vi "Page_Info_Initialize.vi"(8 "error in (no error)":errorcluster, 9 "ctlReferences":T1, 11 "AB_SourceDistribution in":refnum<class "AB_SourceDistribution.lvclass">) -> (0 "error out":errorcluster, 3 "AB_SourceDistribution out":refnum<class "AB_SourceDistribution.lvclass">)   [LabVIEW 2020, in "AB_SourceDistribution.lvclass"]
uses:
  <vilib>/AppBuilder/AB_Classes/SourceDistribution/AB_SourceDistribution.lvclass
  <resource>/Framework/Providers/Builds/AppBuilder/AB_UI_Page_Info_References.ctl
  <resource>/Framework/Providers/Common/provcom_StringGlobals.vi
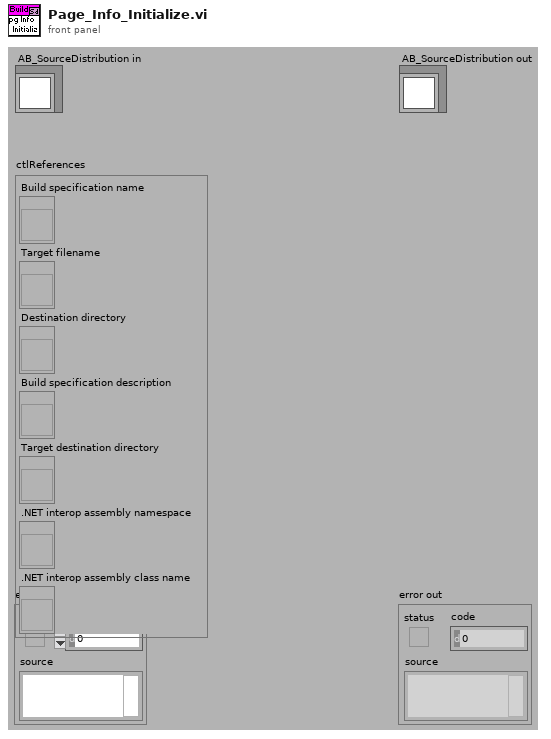
[diagram p1: front panel]
types:
  T1 = typedef "AB_UI_Page_Info_References.ctl" = cluster{"Build specification name":refnum<vi>, "Target filename":refnum<vi>, "Destination directory":refnum<vi>, "Build specification description":refnum<vi>, "Target destination directory":refnum<vi>, ".NET interop assembly namespace":refnum<vi>, ".NET interop assembly class name":refnum<vi>}
  T2 = typedef "LVRectTypeDef.ctl" = cluster{"Left":i16, "Top":i16, "Right":i16, "Bottom":i16}
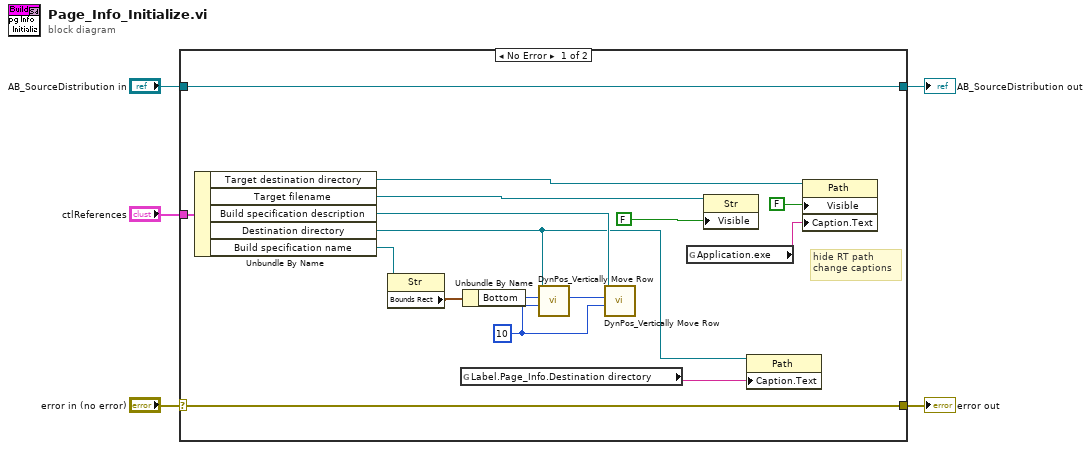
[diagram p0: block diagram]
diagram:
  n1 = case shown="No Error" "error in (no error)" {
    selector: "error in (no error)" -> [w19 w23]
    tunnel: [w19 w23] -> w4
    tunnel: [w20 w22] -> w2
    tunnel: "AB_SourceDistribution in" -> [w20 w22]
    tunnel: "ctlReferences" -> [w21 _]
    frame No Error {
      w14 = 10 ("Pixel separation (6)")
      # "hide RT path\nchange captions"
      n2 = Unbundle By Name(w21) -> ("Target destination directory"=w9:refnum<vi>, "Target filename"=w12:refnum<vi>, "Build specification description"=w13:refnum<vi>, "Destination directory"=w6:refnum<vi>, "Build specification name"=w17:refnum<vi>)
      n3 = property class="Str"(reference=w17) -> ("Bounds Rect"=w18:T2)  [unwired: 1 in, 2 out]
      n4 = global read "provcom_StringGlobals.vi" "Label.Page_Info.Destination directory"() -> (w7:string)
      n5 = Unbundle By Name(w18) -> ("Bottom"=w16:i16)
      n6 = call <vilib>:"DynPos_Vertically Move Row.vi"("Pixel separation (6)"=w14, "Bottom of last control"=w16, "Control"=w6) -> ("Bottom pixel"=w15:i32)  [unwired: 7 in, 1 out]
      n7 = call <vilib>:"DynPos_Vertically Move Row.vi"("Pixel separation (6)"=w14, "Bottom of last control"=w15, "Control"=w13) -> ()  [unwired: 7 in, 2 out]
      n8 = global read "provcom_StringGlobals.vi" "Application.exe"() -> (w8:string)
      n9 = property class="Str"(reference=w12, "Visible"=FALSE) -> ()  [unwired: 1 in, 2 out]
      n10 = property class="Path"(reference=w6, "Caption.Text"=w7) -> ()  [unwired: 1 in, 2 out]
      n11 = property class="Path"(reference=w9, "Visible"=FALSE, "Caption.Text"=w8) -> ()  [unwired: 1 in, 2 out]
    }
    frame Error {
    }
  }
  "error out" <- w4
  "AB_SourceDistribution out" <- w2
